vi "Remove Elements from Array by Index.vi"(1 "Indices":i32[](array[numeric]), 2 "Array In":dbl[](array[numeric])) -> (0 "Array Out 2":dbl[](array[numeric]))   [LabVIEW 2020]
doc: "Remove Elements from Array by Index.vi takes an integer array as input and removes all elements of an inputted double numeric array with the inputted indices."
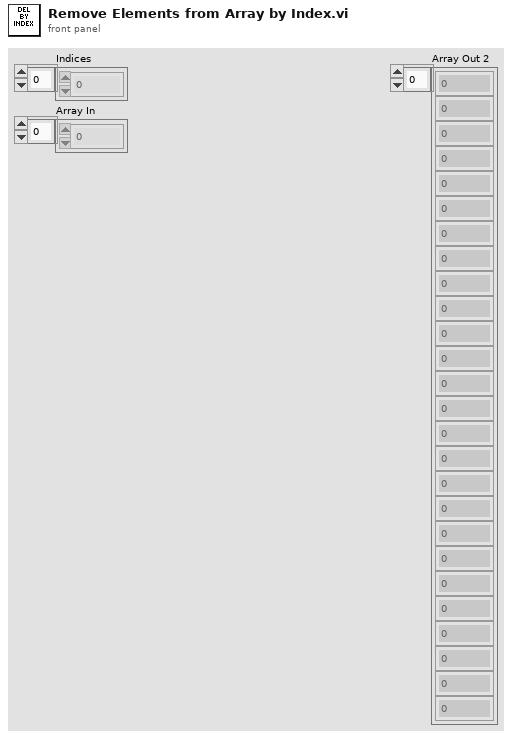
[diagram p1: front panel]
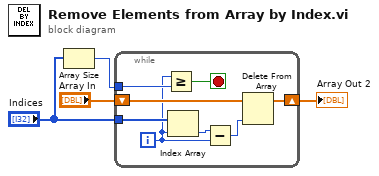
[diagram p0: block diagram]
diagram:
  n1 = Array Size(array="Indices") -> (size(s)=w4:i32)
  n2 = while {
    tunnel: w4 -> [w12]
    tunnel: "Indices" -> [w9]
    shift-right: [w8] -> w1
    shift-left: "Array In" -> [w10]
    i -> [w6]
    stop <- w11 stop-if-true
    n3 = Greater Or Equal?(x=w6, y=w12) -> (x >= y?=w11:bool)
    n4 = Index Array(array=w9, index=w6) -> (element=w7:i32)
    n5 = Subtract(x=w7, y=w6) -> (x-y=w5:i32)
    n6 = Delete From Array(array=w10, index=w5) -> (array with subset deleted=w8:dbl[])  [unwired: 1 in, 1 out]
  }
  "Array Out 2" <- w1
